vi "getSheetData.vi"(0 "reference in":refnum<class "python.lvclass">, 1 "filePath":string, 2 "sheetName":string, 3 "column":string, 4 "row":string, 5 "error in (no error)":errorcluster) -> (14 "reference out":refnum<class "python.lvclass">, 16 "dataOut":string[][](array[string]), 19 "error out":errorcluster)   [LabVIEW 2016, in "python.lvclass"]
uses:
  python.lvclass
  <vilib>/Utility/error.llb/DialogType.ctl
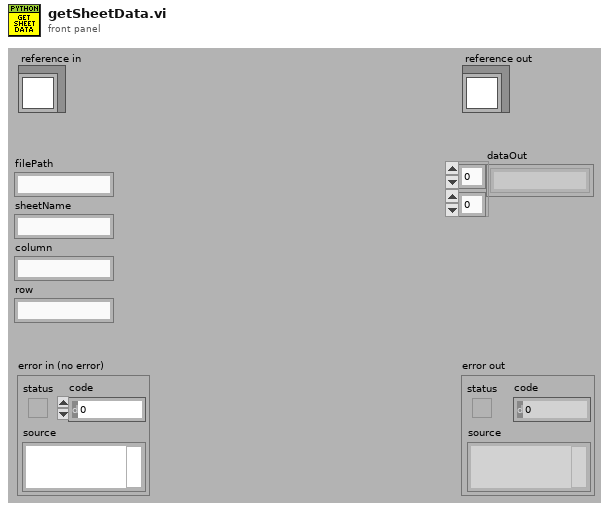
[diagram p1: front panel]
types:
  T1 = typedef "python.lvclass/ObjectAttributesRef.ctl" = refnum<data-value>
  T2 = typedef "python.lvclass/ObjectAttributes.ctl" = cluster{"MyAttribute":dbl, "workingDirectory":path}
  T3 = typedef "DialogType.ctl" = u16
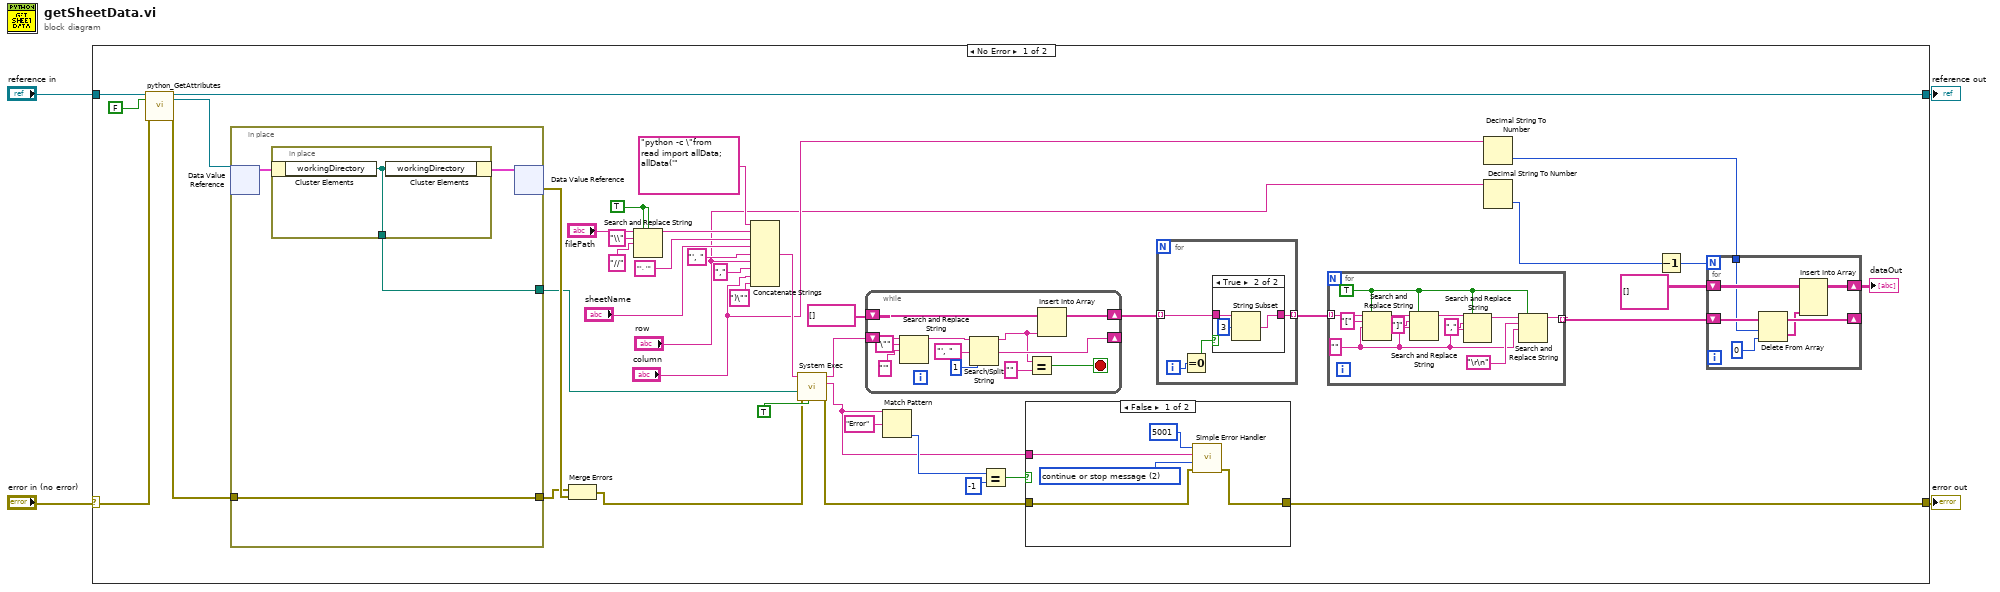
[diagram p0: block diagram]
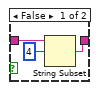
[diagram p2: hidden frame]
diagram:
  n1 = case shown="No Error" "error in (no error)" {
    selector: "error in (no error)" -> [w42 w99]
    tunnel: [w31 w99] -> w3
    tunnel: [w40 w98] -> w1
    tunnel: "reference in" -> [w44 w98]
    frame No Error {
      w26 = TRUE ("replace all? (F)")
      n2 = call "python_GetAttributes.vi"("reference in"=w44, "return data? (T)"=FALSE, "error in (no error)"=w42) -> ("reference out"=w40:refnum<class "python.lvclass">, "attributes ref"=w39:T1, "error out"=w41:errorcluster)  [unwired: 13 in, 1 out]
      n3 = in-place {
        in-place-border: w41 -> [w94]
        in-place-border: [w94] -> w45
        in-place-border: [w93] -> w37
        n4 = in-place-dvr #1(w39) -> (w95:T2)  [unwired: 1 out]
        n5 = in-place {
          in-place-border: [w97] -> w93
          n6 = in-place-cluster #2(w95) -> ("workingDirectory"=w97:path)
          n7 = in-place-cluster #2("workingDirectory"=w97) -> (w96:T2)
        }
        n8 = in-place-dvr #1(w96) -> (w46:errorcluster)  [unwired: 1 out]
      }
      n9 = Merge Errors(w45, w46) -> (w36:errorcluster)
      n10 = Search and Replace String(replace all?=w26, case sensitive?=w26, input string="filePath", search string="\\", replace string="//" ("search string")) -> (result string=w27:string)  [unwired: 3 in, 3 out]
      n11 = Concatenate Strings("python -c \"from read import allData; allData('" ("string"), w27, "', '" ("string"), "sheetName", "', " ("string"), "row", "," ("string"), "column", ")\"" ("string")) -> (w33:string)
      n12 = call <vilib>:"System Exec.vi"("run minimized? (F)"=TRUE, "error in (no error)"=w36, "working directory"=w37, "command line"=w33) -> ("error out"=w32:errorcluster, "standard error"=w12:string, "standard output"=w13:string)  [unwired: 2 in, 3 out]
      n13 = while {
        shift-right: [w85] -> w15
        shift-left: string[] [] -> [w86]
        shift-right: [w84] -> _
        shift-left: w13 -> [w78]
        stop <- w83 stop-if-true
        n14 = Search and Replace String(input string=w78, search string="\"", replace string="'" ("replace string (\"\")")) -> (result string=w77:string)  [unwired: 5 in, 3 out]
        n15 = Search/Split String(string=w77, search string/char (-)="', ", offset (0)=1) -> (substring before match=w81:string, match + rest of string=w84:string)  [unwired: 1 out]
        n16 = Equal?(x=w81, y="") -> (x = y?=w83:bool)
        n17 = Insert Into Array(array=w86, new element=w81) -> (w85:string[])  [unwired: 1 in]
      }
      n18 = Match Pattern(string=w12, regular expression="Error") -> (offset past match=w22:i32)  [unwired: 1 in, 3 out]
      n19 = Equal?(x=w22, y=-1 ("offset past match")) -> (x = y?=w23:bool)
      n20 = case shown="False" w23 {
        tunnel: w32 -> [w91 w92]
        tunnel: [w90 w92] -> w31
        tunnel: w12 -> [w88 _]
        frame False {
          w87 = T3 2 items=["no dialog", "OK message", "continue or stop message", "OK message + warnings", "continue/stop + warnings"] ("type of dialog (OK msg:1)")
          n21 = call <vilib>:"Simple Error Handler.vi"("error code (no error:0)"=5001, "error source (\" \")"=w88, "type of dialog (OK msg:1)"=w87, "error in (no error)"=w91) -> ("error out"=w90:errorcluster)  [unwired: 5 out]
        }
        frame True {
        }
      }
      n22 = for {
        tunnel: w15 -> [w50] mode=indexing
        tunnel: [w49] -> w14 mode=indexing
        i -> [w48]
        n23 = Equal To 0?(x=w48) -> (x = 0?=w47:bool)
        n24 = case shown="True" w47 {
          tunnel: w50 -> [w53 w56]
          tunnel: [w51 w55] -> w49
          frame False {
            n25 = String Subset(string=w53, offset (0)=4) -> (substring=w51:string)  [unwired: 1 in]
          }
          frame True {
            n26 = String Subset(string=w56, offset (0)=3) -> (substring=w55:string)  [unwired: 1 in]
          }
        }
      }
      n27 = for {
        tunnel: w14 -> [w74] mode=indexing
        tunnel: [w66] -> w17 mode=indexing
        w67 = TRUE ("replace all? (F)")
        w68 = "" ("replace string (\"\")")
        n28 = Search and Replace String(replace all?=w67, input string=w74, search string="[", replace string=w68) -> (result string=w72:string)  [unwired: 4 in, 3 out]
        n29 = Search and Replace String(replace all?=w67, input string=w72, search string="]", replace string=w68) -> (result string=w65:string)  [unwired: 4 in, 3 out]
        n30 = Search and Replace String(replace all?=w67, input string=w65, search string=",", replace string=w68) -> (result string=w64:string)  [unwired: 4 in, 3 out]
        n31 = Search and Replace String(replace all?=w67, input string=w64, search string="\r\n", replace string=w68) -> (result string=w66:string)  [unwired: 4 in, 3 out]
      }
      n32 = Decimal String To Number(string="column") -> (number=w8:i32)  [unwired: 2 in, 1 out]
      n33 = Decimal String To Number(string="row") -> (number=w10:i32)  [unwired: 2 in, 1 out]
      n34 = Decrement(x=w10) -> (x-1=w9:i32)
      n35 = for {
        N: w9 -> [_]
        shift-right: [w61] -> w11
        shift-left: string[][] [] -> [w62]
        shift-right: [w60] -> _
        shift-left: w17 -> [w63]
        tunnel: w8 -> [w58]
        n36 = Delete From Array(array=w63, length=w58, index=0) -> (deleted portion=w57:string[], array with subset deleted=w60:string[])
        n37 = Insert Into Array(array=w62, new element=w57) -> (w61:string[][])  [unwired: 2 in]
      }
      "dataOut" <- w11
    }
    frame Error {
    }
  }
  "error out" <- w3
  "reference out" <- w1
